vi "PPL Paths.vi"() -> (1 "Install PPL":path, 2 "Shipped Backup":path, 3 "Current PPL":path)   [LabVIEW 2021]
doc: "Returns the paths of the PPLs and what they should be renamed to."
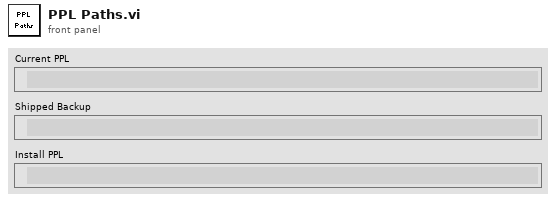
[diagram p1: front panel]
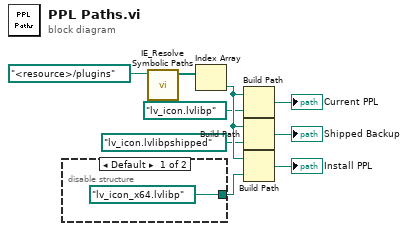
[diagram p0: block diagram]
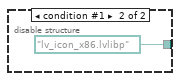
[diagram p2: hidden frame]
diagram:
  n1 = disable-structure shown="Default" {
    disable-tunnel: [path "lv_icon_x64.lvlibp" ("name or relative path") path "lv_icon_x86.lvlibp" ("name or relative path")] -> w5
    frame condition #0 (active) {
    }
    frame condition #1 {
    }
  }
  n2 = call <resource>:"IE_Resolve Symbolic Paths.vi"("symbolic path"=path "<resource>/plugins") -> ("resolved paths"=w1:path[])  [unwired: 10 in]
  n3 = Index Array(array=w1) -> (element=w9:path)  [unwired: 1 in]
  n4 = Build Path(base path=w9, name or relative path=path "lv_icon.lvlibp") -> (appended path=→"Current PPL":path)
  n5 = Build Path(base path=w9, name or relative path=path "lv_icon.lvlibpshipped") -> (appended path=→"Shipped Backup":path)
  n6 = Build Path(base path=w9, name or relative path=w5) -> (appended path=→"Install PPL":path)
